vi "Untitled 1.vi"() -> ()   [LabVIEW 2013]
panel:
  out "Slide 2":dbl(slide) scale=1.0..6.0
  in  "Hit Limit?":bool
  in  "Desired Position":i32
  out "Slide":dbl(slide) scale=-1.0..1.0
  in  "Right":bool
  in  "Left":bool
  out "Indicator":bool
  in  "Length Of Blinks":dbl
  in  "Time In Between Blinks":dbl
  in  "Number of Blinks":dbl
  in  "Input":bool
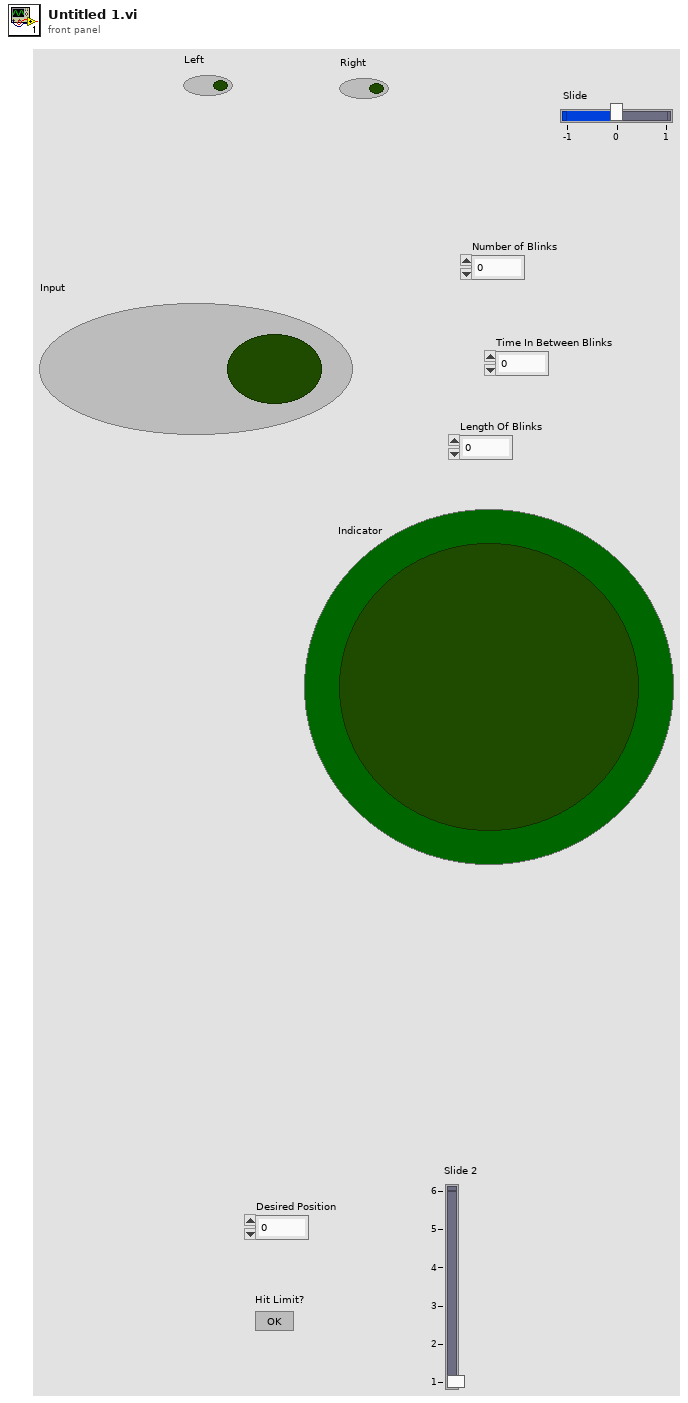
[diagram p1: front panel]
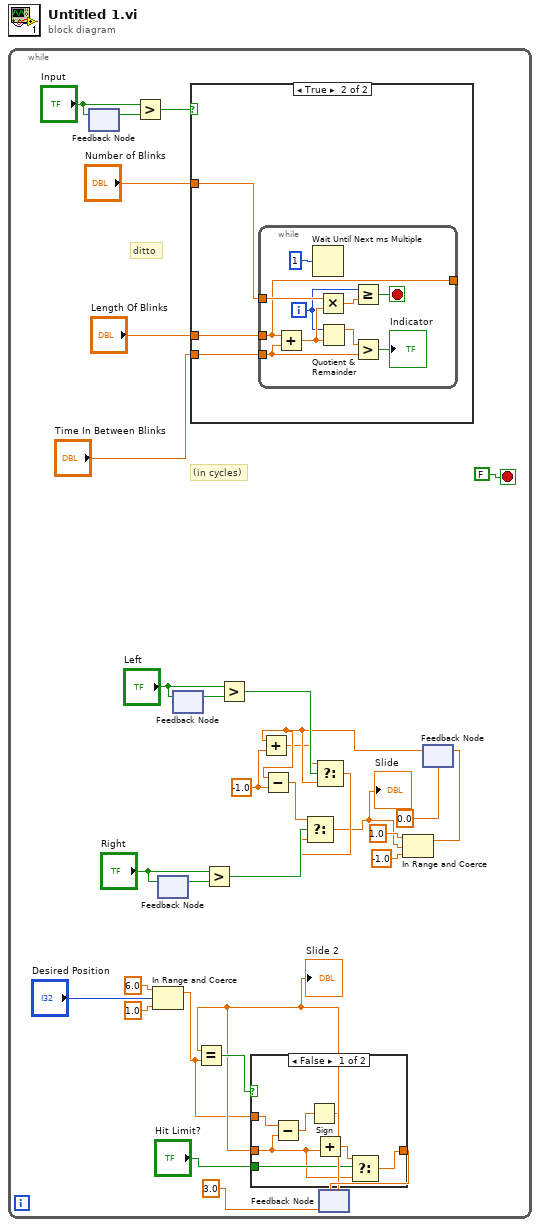
[diagram p0: block diagram]
diagram:
  n1 = while {
    stop <- FALSE stop-if-true
    w17 = -1.0 ("y")
    # "ditto"
    # "(in cycles)"
    n2 = feedback-in #1("Input") -> ()
    n3 = feedback #1() -> (w30:bool)  [unwired: 1 in]
    n4 = Greater?(x="Input", y=w30) -> (0:w26:bool)
    n5 = In Range and Coerce(upper limit=6.0, x="Desired Position", lower limit=1.0) -> (coerced(x)=w1:dbl)  [unwired: 1 out]
    n6 = feedback #2() -> (w24:bool)  [unwired: 1 in]
    n7 = feedback-in #2("Right") -> ()
    n8 = feedback #3() -> (w25:bool)  [unwired: 1 in]
    n9 = feedback-in #3("Left") -> ()
    n10 = case shown="True" w26 {
      tunnel: "Length Of Blinks" -> [_ w41]
      tunnel: "Time In Between Blinks" -> [_ w42]
      tunnel: "Number of Blinks" -> [_ w43]
      frame False {
      }
      frame True {
        n11 = while {
          tunnel: w42 -> [w48]
          tunnel: [w44] -> _
          tunnel: w43 -> [w52]
          tunnel: w41 -> [w44]
          i -> [w46]
          stop <- w51 stop-if-true
          n12 = Add(x=w44, y=w48) -> (x+y=w50:dbl)
          n13 = Wait Until Next ms Multiple(millisecond multiple=u32 1) -> ()  [unwired: 1 out]
          n14 = Multiply(x=w52, y=w50) -> (x*y=w47:dbl)
          n15 = Quotient & Remainder(x=w46, y=w50) -> (x-y*floor(x/y)=w49:dbl)  [unwired: 1 out]
          n16 = Greater Or Equal?(x=w46, y=w47) -> (x >= y?=w51:bool)
          n17 = Greater?(x=w49, y=w48) -> (0:→"Indicator":bool)
        }
      }
    }
    n18 = Greater?(x="Right", y=w24) -> (0:w16:bool)
    n19 = Greater?(x="Left", y=w25) -> (0:w15:bool)
    n20 = feedback #4(3.0 ("upper limit")) -> (w3:dbl)
    "Slide 2" <- w3
    n21 = Equal?(x=w3, y=w1) -> (x = y?=w5:bool)
    n22 = case shown="False" w5 {
      tunnel: w3 -> [w34 w40]
      tunnel: [w33 w40] -> w4
      tunnel: "Hit Limit?" -> [w35 _]
      tunnel: w1 -> [w38 _]
      frame False {
        n23 = Subtract(x=w38, y=w34) -> (x-y=w37:dbl)
        n24 = Sign(1:w37) -> (0:w39:dbl)
        n25 = Add(x=w39, y=w34) -> (x+y=w36:dbl)
        n26 = Select(t=w36, s=w35, f=w34) -> (s? t:f=w33:dbl)
      }
      frame True {
      }
    }
    n27 = feedback-in #4(w4) -> ()
    n28 = feedback #5(0.0 ("upper limit")) -> (w14:dbl)
    n29 = Add(x=w14, y=w17) -> (x+y=w13:dbl)
    n30 = Subtract(x=w14, y=w17) -> (x-y=w11:dbl)
    n31 = Select(t=w13, s=w15, f=w14) -> (s? t:f=w12:dbl)
    n32 = Select(t=w11, s=w16, f=w12) -> (s? t:f=w10:dbl)
    "Slide" <- w10
    n33 = In Range and Coerce(upper limit=1.0, x=w10, lower limit=-1.0) -> (coerced(x)=w19:dbl)  [unwired: 1 out]
    n34 = feedback-in #5(w19) -> ()
  }
